vi "AndorLiveMode.vi"(8 "error in (no error)":errorcluster, 11 "Image Name":string="untitled") -> (0 "error out":errorcluster, 3 "Image":T1(plugin-control))   [LabVIEW 2018]
uses:
  <vilib>/vision/NI_Vision_Development_Module.lvlib
  <userlib>/Andor SDK/Andor SDK.lvlib
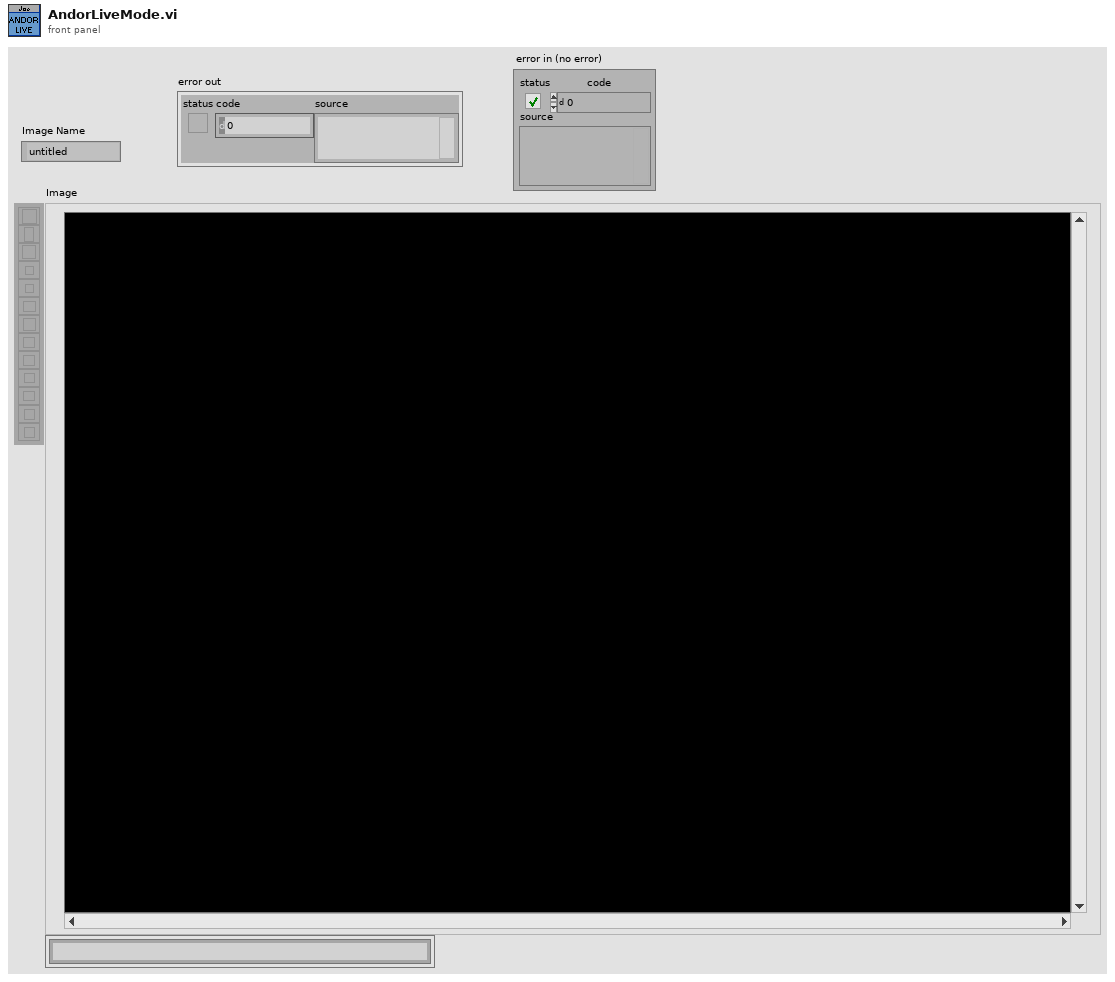
[diagram p1: front panel]
types:
  T1 = typedef "IMAQ Image.ctl" = refnum<image>
  T2 = typedef "Image Type" = u32
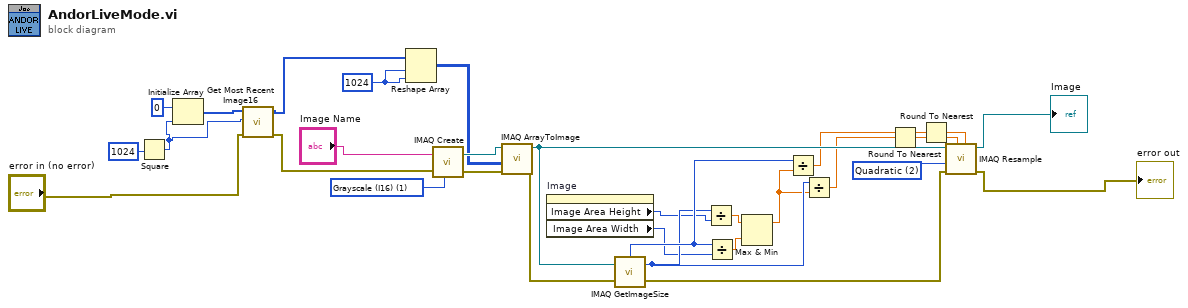
[diagram p0: block diagram]
diagram:
  w14 = u32 2 items=["Zero Order", "Bi-Linear", "Quadratic", "Cubic Spline"] ("Interpolation Type")
  w26 = T2 1 items=["Grayscale (U8)", "Grayscale (I16)", "Grayscale (SGL)", "Complex (CSG)", "RGB (U32)", "HSL (U32)", "RGB (U64)", "Grayscale (U16)"] ("Image Type")
  w27 = 1024 ("dimension size")
  n1 = Square(x=1024) -> (x^2=w4:i32)
  n2 = Initialize Array(0 ("element"), w4) -> (w5:i32[])
  n3 = call <userlib>:"Get Most Recent Image16.vi"("error in (no error)"="error in (no error)", "size"=w4, "arr"=w5) -> ("error out"=w1:errorcluster, "arr out"=w3:u16[])  [unwired: 6 in, 1 out]
  n4 = Reshape Array(w3, w27, w27) -> (w23:u16[][])
  n5 = call "IMAQ Create"("Image Name"="Image Name", "Image Type"=w26, "error in (no error)"=w1) -> ("New Image"=w25:T1, "error out"=w24:errorcluster)  [unwired: 2 in]
  n6 = call "IMAQ ArrayToImage"("error in (no error)"=w24, "Image Pixels (I16)"=w23, "Image"=w25) -> ("error out"=w20:errorcluster, "Image Out"=w16:T1)  [unwired: 7 in]
  n7 = property on="Image" class="ImageControl"() -> ("Image Area Height"=w10:u32, "Image Area Width"=w13:u32)  [unwired: 2 in, 2 out]
  n8 = call "IMAQ GetImageSize"("Image"=w16, "error in (no error)"=w20) -> ("Y Resolution"=w18:i32, "X Resolution"=w19:i32, "error out"=w15:errorcluster)  [unwired: 2 in]
  n9 = Divide(x=w18, y=w10) -> (x/y=w22:dbl)
  n10 = Divide(x=w19, y=w13) -> (x/y=w21:dbl)
  n11 = Max & Min(x=w22, y=w21) -> (max(x,y)=w17:dbl)  [unwired: 1 out]
  n12 = Divide(x=w19, y=w17) -> (x/y=w8:dbl)
  n13 = Divide(x=w18, y=w17) -> (x/y=w9:dbl)
  n14 = Round To Nearest(number=w9) -> (nearest integer value=w6:dbl)
  n15 = Round To Nearest(number=w8) -> (nearest integer value=w7:dbl)
  n16 = call "IMAQ Resample"("X Resolution"=w7, "Y Resolution"=w6, "error in (no error)"=w15, "Interpolation Type"=w14, "Image Src"=w16) -> ("error out"=→"error out":errorcluster, "Image Dst Out"=→"Image":T1)  [unwired: 5 in]
